vi "TrimShortcutPrefix.vi"(0 "String in":string) -> (14 "String out":string)   [LabVIEW 2017, in "NEVSTOP QD Shortcuts.lvlib"]
uses:
  NEVSTOP QD Shortcuts.lvlib
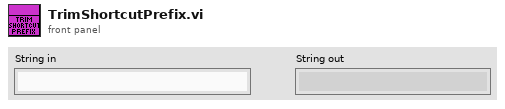
[diagram p1: front panel]
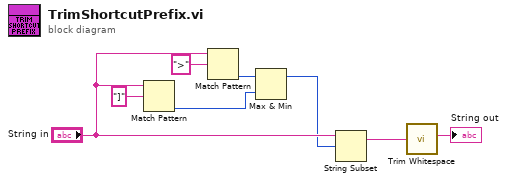
[diagram p0: block diagram]
diagram:
  n1 = Match Pattern(string="String in", regular expression="]") -> (offset past match=w2:i32)  [unwired: 1 in, 3 out]
  n2 = Match Pattern(string="String in", regular expression=">") -> (offset past match=w3:i32)  [unwired: 1 in, 3 out]
  n3 = Max & Min(x=w3, y=w2) -> (max(x,y)=w1:i32)  [unwired: 1 out]
  n4 = String Subset(string="String in", offset (0)=w1) -> (substring=w8:string)  [unwired: 1 in]
  n5 = call-poly <vilib>:"Trim Whitespace.vi"("string"=w8) -> ("trimmed string"=→"String out":string)  [unwired: 1 in]
